vi "preConfigCreate.vi"(7 "Shared Resource (F)":bool, 8 "error in (no error)":errorcluster, 10 "Subsystem Name (optional)":string, 11 "SMO in":refnum<class "SMO.lvclass">) -> (0 "error out":errorcluster, 3 "SMO out":refnum<class "SMO.lvclass">)   [LabVIEW 2013, in "SMO.lvclass"]
uses:
  SMO.lvclass
  Registry/Registry-SMO.lvclass
  Support/Attribute.Dependencies/Attribute.Dependencies.lvclass
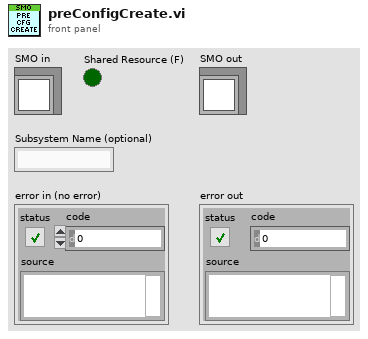
[diagram p1: front panel]
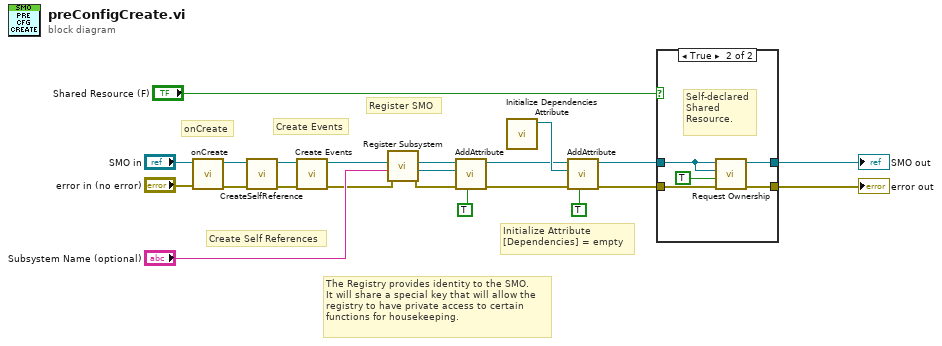
[diagram p0: block diagram]
diagram:
  # "Initialize Attribute\n[Dependencies] = empty"
  # "The Registry provides identity to the SMO.\nIt will share a special key that will allow the\nregistry to have private access to certain\nfunctions for housekeeping."
  # "Create Self References"
  # "Register SMO"
  # "Create Events"
  # "onCreate"
  n1 = call-dynamic "onCreate.vi"("error in (no error)"="error in (no error)", "SMO"="SMO in") -> ("error out"=w15:errorcluster, "SMO out"=w13:refnum<class "SMO.lvclass">)  [unwired: 8 in]
  n2 = call-dynamic "CreateSelfReference.vi"("error in (no error)"=w15, "SMO"=w13) -> ("error out"=w16:errorcluster, "SMO out"=w14:refnum<class "SMO.lvclass">)  [unwired: 8 in]
  n3 = call "Create Events.vi"("error in (no error)"=w16, "SMO"=w14) -> ("error out"=w7:errorcluster, "SMO out"=w6:refnum<class "SMO.lvclass">)  [unwired: 8 in]
  n4 = call "Register Subsystem.vi"("error in (no error)"=w7, "Subsystem Name (optional)"="Subsystem Name (optional)", "Unregistered SMO"=w6) -> ("error out"=w12:errorcluster, "Attribute.Identity"=w17:refnum<class "Attribute.Identity.lvclass">, "Registered SMO"=w11:refnum<class "SMO.lvclass">)  [unwired: 6 in]
  n5 = call "AddAttribute.vi"("Overwrite? (F)"=TRUE, "error in (no error)"=w12, "Attribute"=w17, "SMO in"=w11) -> ("error out"=w21:errorcluster, "SMO out"=w18:refnum<class "SMO.lvclass">)  [unwired: 6 in]
  n6 = call "Initialize Dependencies Attribute.vi"() -> ("Attribute.Dependencies"=w19:refnum<class "Attribute.Dependencies.lvclass">)  [unwired: 11 in]
  n7 = call "AddAttribute.vi"("Overwrite? (F)"=TRUE, "error in (no error)"=w21, "Attribute"=w19, "SMO in"=w18) -> ("error out"=w4:errorcluster, "SMO out"=w2:refnum<class "SMO.lvclass">)  [unwired: 6 in]
  n8 = case shown="True" "Shared Resource (F)" {
    tunnel: [w24 w29] -> w1
    tunnel: w4 -> [w23 w28]
    tunnel: [w23 w27] -> w3
    tunnel: w2 -> [w24 w26]
    frame False {
    }
    frame True {
      # "Self-declared\nShared\nResource."
      n9 = call "Request Ownership.vi"("error in (no error)"=w28, "Shared Resource"=TRUE, "Dependency"=w26, "SMO in"=w26) -> ("error out"=w27:errorcluster, "SMO out"=w29:refnum<class "SMO.lvclass">)  [unwired: 5 in, 1 out]
    }
  }
  "error out" <- w3
  "SMO out" <- w1
